vi "Write.Initialize.vi"(8 "error in (no error)":errorcluster, 11 "Write in":refnum<class "Write.lvclass">) -> (0 "error out":errorcluster, 3 "Write out":refnum<class "Write.lvclass">)   [LabVIEW 2015, in "Data Access API.lvlib" / "Write.lvclass"]
uses:
  Write.lvclass
  Write.lvclass/Write.ctl
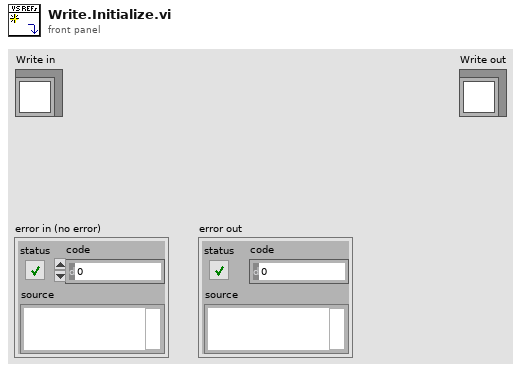
[diagram p1: front panel]
types:
  T1 = cluster{"read mode":enum16{"polling", "blocking"}, "write mode":enum16{"polling", "blocking"}}
  T2 = typedef "Custom Device API.lvlib/Data Reference.ctl" = i32
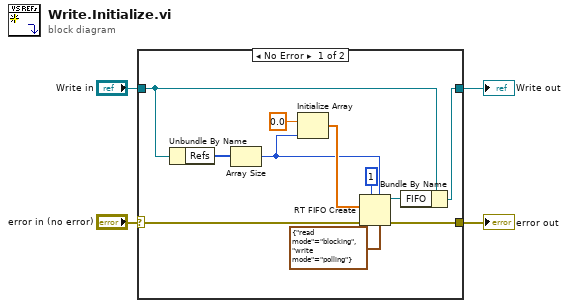
[diagram p0: block diagram]
diagram:
  n1 = case shown="No Error" "error in (no error)" {
    selector: "error in (no error)" -> [w5 w16]
    tunnel: [w15 w16] -> w4
    tunnel: "Write in" -> [w7 w17]
    tunnel: [w6 w17] -> w2
    frame No Error {
      n2 = Unbundle By Name(w7) -> ("Refs"=w8:T2[])
      n3 = Array Size(array=w8) -> (size(s)=w10:i32)
      n4 = Initialize Array(0.0 ("element"), w10) -> (w13:dbl[])
      n5 = RT FIFO Create(1:w13, 3:w5, 4:u32 1 ("size (10)"), 6:w10, 7:T1 {"read mode"=enum."blocking", "write mode"=enum."polling"} ("r/w modes (polling,polling)")) -> (8:w14:refnum<k33>, 11:w15:errorcluster)  [unwired: 3 in, 1 out]
      n6 = Bundle By Name(cluster=w7, "FIFO"=w14) -> (w6:refnum<class "Write.lvclass">)
    }
    frame Error {
    }
  }
  "error out" <- w4
  "Write out" <- w2
